vi "G_ALL.vi"() -> ()   [LabVIEW 2015]
panel:
  out "xym 4":dbl[][](array[numeric])
  out "xym 3":dbl[][](array[numeric])
  out "xym 2":dbl[][](array[numeric])
  out "xym 1":dbl[][](array[numeric])
  out "mission num":i32
  out "mission":dbl[](array[numeric])
  out "curve vel limit":dbl=-3.32529799262397
  out "Avante_shift":u8
  out "dist lane":dbl[](array[numeric])
  out "map_track lane":dbl[][](array[numeric])
  out "map_track 2":dbl[][](array[numeric])
  out "v origin":dbl[](array[numeric])
  out "current idx":i32
  out "dist":dbl[](array[numeric])
  out "heading":dbl[](array[numeric])
  in  "OBS":bool
  out "Steering":dbl=-3.32529799262397
  out "VS_des":dbl=30.0
  in  "replay":bool
  in  "Reverse":bool
  in  "E-STOP":bool
  out "file path":path
  out "x_ibeo":cluster{"idx":i32, "x":dbl, "y":dbl, "h":dbl}={"idx"=1, "x"=-35.60561147, "y"=-90.69379038, "h"=0.8330275943157105}
  out "CARCONTROL":cluster{"speed path":dbl, "speed limit":dbl}={"speed path"=30.0, "speed limit"=2.65}
  out "beep":T1={"beep"=FALSE, "duration (msec)"=100, "frequency (Hz)"=1200}
  out "CARSPEC":T2={"C_Wheel base"=2.65, "ratio_steer"=15.6, "Overall width"=2.65, "af"=2.65, "turn radius"=5.50164, "eval"=0.1, "ap"=2.777777777777778, "an"=-1.736111111111111, "Vmax"=200.0, "mu"=0.15, "Vlast"=200.0}
  out "xobs":cluster{"idx":i32, "x":dbl, "y":dbl, "h":dbl}
  in  "ecef ref":dbl[](array[numeric]) format="%#_19f"
  out "map_track_saved":dbl[][](array[numeric])
  out "map_track":dbl[][](array[numeric])
  out "y origin":dbl[](array[numeric])
  out "x origin":dbl[](array[numeric])
  out "GPSDATA":T3={"hash"=1114363806672425932, "sys time"=0, "time"=0.0, "x"=0.0, "y"=0.0, "h"=0.0, "numSV"=0, "postype"=0, "lag"=0, "hordev"=0.0, "lat"=0.0, "lon"=0.0, "hgt"=0.0, "map_idx"=0} {"hash" format="%016x"}
  out "CARDATA":T4={"Steer_input"=-119.00362066056654, "Steer_output"=-0.0, "VS_des"=0.0, "VS_can"=0.0, "heading"=0.0, "auto"=FALSE, "run"=FALSE, "x"=0.0, "y"=0.0}
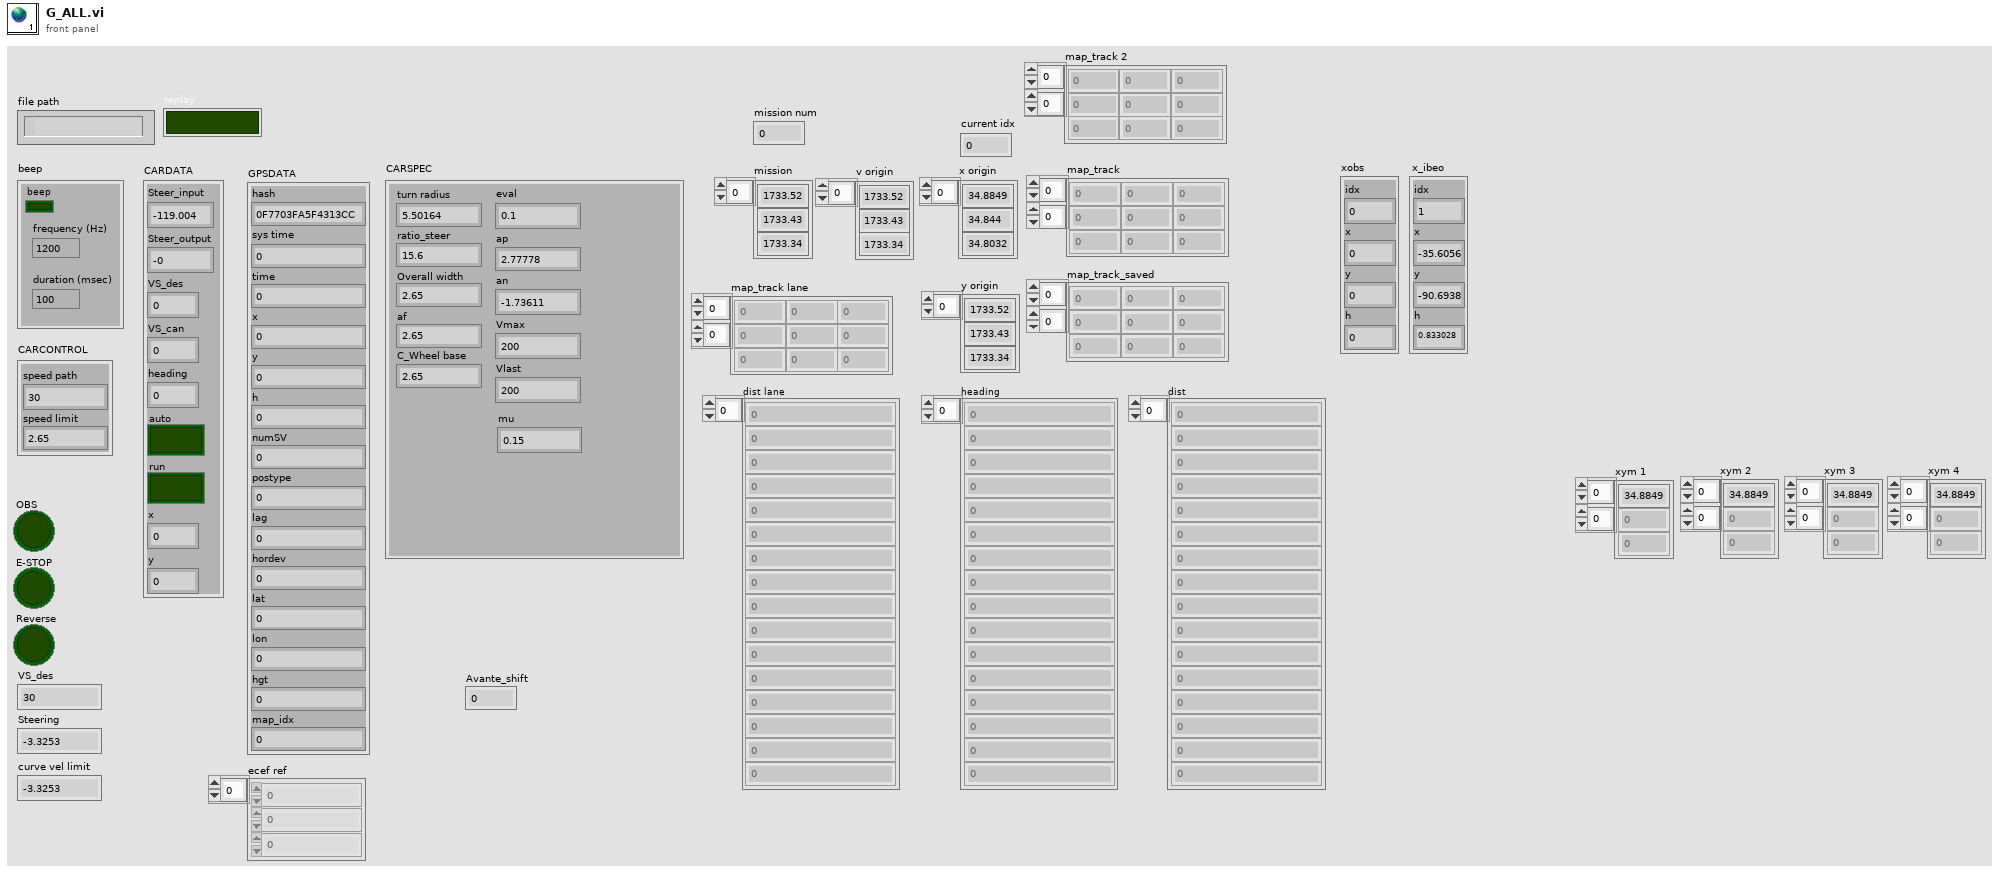
[diagram p1: front panel]
types:
  T1 = cluster{"beep":bool, "duration (msec)":u32, "frequency (Hz)":u32}
  T2 = cluster{"C_Wheel base":dbl, "ratio_steer":dbl, "Overall width":dbl, "af":dbl, "turn radius":dbl, "eval":dbl, "ap":dbl, "an":dbl, "Vmax":dbl, "mu":dbl, "Vlast":dbl}
  T3 = cluster{"hash":i64, "sys time":i64, "time":dbl, "x":dbl, "y":dbl, "h":dbl, "numSV":i32, "postype":i32, "lag":i32, "hordev":dbl, "lat":dbl, "lon":dbl, "hgt":dbl, "map_idx":i32}
  T4 = cluster{"Steer_input":dbl, "Steer_output":dbl, "VS_des":dbl, "VS_can":dbl, "heading":dbl, "auto":bool, "run":bool, "x":dbl, "y":dbl}
diagram:
